vi "Read Word From 2 Addresses.vi"(8 "Error in (no error)":errorcluster, 9 "Address number (0)":u8, 10 "Motor ID (0)":u8, 11 "VISA resource name":refnum<visa-resource-name>) -> (0 "error out":errorcluster, 2 "Data":u16, 3 "VISA resource name out":refnum<visa-resource-name>)   [LabVIEW 2016, in "Dynamixel Motor.lvlib"]
doc: "Reads a word type (U16) from two addresses of a Dynamixel motor. The value returned will typically range from 0 to 1023. This VI assumes little endian byte order. This is a Low-Level VI that is used by other VIs."
uses:
  Dynamixel Motor.lvlib
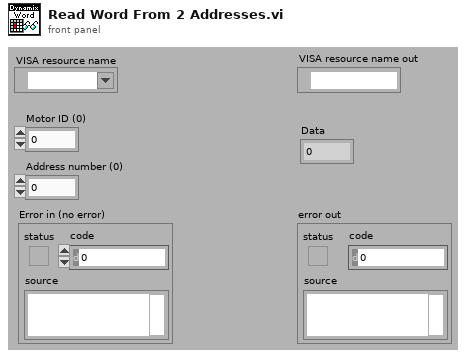
[diagram p1: front panel]
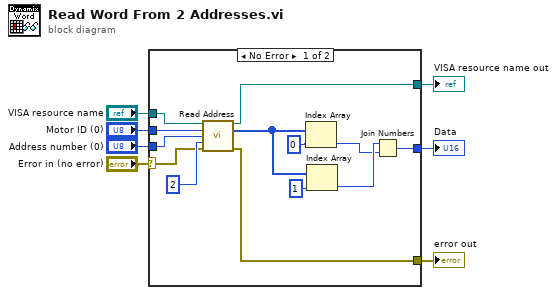
[diagram p0: block diagram]
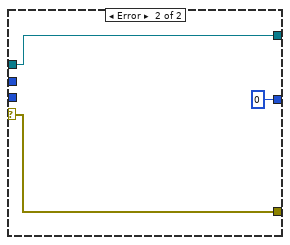
[diagram p2: hidden frame]
diagram:
  n1 = case shown="No Error" "Error in (no error)" {
    selector: "Error in (no error)" -> [w11 w23]
    tunnel: [w8 u16 0] -> w7
    tunnel: "VISA resource name" -> [w17 w22]
    tunnel: [w16 w22] -> w5
    tunnel: [w15 w23] -> w4
    tunnel: "Address number (0)" -> [w13 _]
    tunnel: "Motor ID (0)" -> [w12 _]
    frame No Error {
      n2 = call "Read Address.vi"("VISA resource name"=w17, "Motor ID (0)"=w12, "Address number (0)"=w13, "Number of Addresses to read (1)"=u8 2, "Error in (no error)"=w11) -> ("VISA resource name Out"=w16:refnum<visa-resource-name>, "Data Read"=w20:u8[], "error out"=w15:errorcluster)  [unwired: 7 in, 1 out]
      n3 = Index Array(array=w20, index=0) -> (element=w9:u8)
      n4 = Index Array(array=w20, index=1) -> (element=w10:u8)
      n5 = Join Numbers(hi=w10, lo=w9) -> ((hi.lo)=w8:u16)
    }
    frame Error {
    }
  }
  "Data" <- w7
  "VISA resource name out" <- w5
  "error out" <- w4
